vi "Set me as Bearer.vi"(8 "error in":errorcluster, 11 "Guardian in":refnum<class "Guardian.lvclass">) -> (0 "error out":errorcluster, 3 "Guardian out":refnum<class "Guardian.lvclass">)   [LabVIEW 2026, in "TALOS.lvlib" / "Guardian.lvlib" / "Guardian.lvclass"]
uses:
  Guardian.lvclass
  C:/LabVIEW Code/TALOS/talos/Ancestor/Ancestor/Ancestor.lvclass
  Ancestor/Ancestor/Ancestor.lvclass/Ancestor.ctl
  Guardian.lvclass/Guardian.ctl
  Ancestor/Ancestor/Ancestor.lvclass
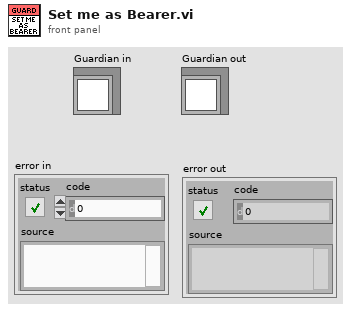
[diagram p1: front panel]
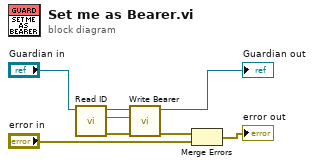
[diagram p0: block diagram]
diagram:
  n1 = call "Read ID.vi"("Ancestor in"="Guardian in") -> ("error out"=w7:errorcluster, "ID"=w6:string, "Ancestor out"=w4:refnum<class "Guardian.lvclass">)  [unwired: 8 in]
  n2 = call "Write Bearer.vi"("error in (no error)"=w7, "Bearer"=w6, "Guardian in"=w4) -> ("error out"=w8:errorcluster, "Guardian out"=→"Guardian out":refnum<class "Guardian.lvclass">)  [unwired: 7 in]
  n3 = Merge Errors(w8, "error in") -> (→"error out":errorcluster)
